vi "串口发送.vi"() -> ()   [LabVIEW 2017]
uses:
  <vilib>/Instr/_visa.llb/VISA Flush IO Buffer Mask.ctl
  <vilib>/Instr/_visa.llb/VISA Configure Serial Port (Instr).vi
panel:
  out "波形图表":dbl(graph)
  in  "停止":bool
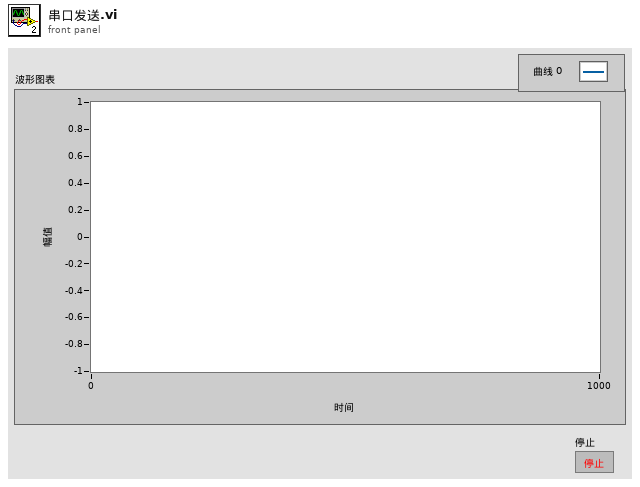
[diagram p1: front panel]
types:
  T1 = typedef "VISA Flush IO Buffer Mask.ctl" = u16
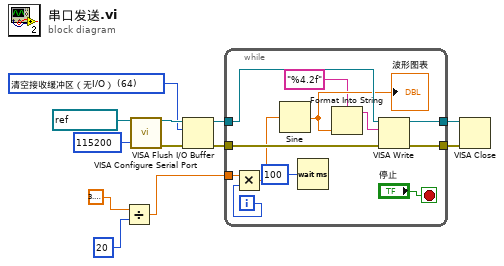
[diagram p0: block diagram]
diagram:
  w8 = T1 64 items=["清空接收缓冲区"=16, "向设备写入传输缓冲区"=32, "清空接收缓冲区（无I/O）"=64, "清空传输缓冲区"=128] ("Mask")
  n1 = Divide(x=3.141592653589793, y=20) -> (x/y=w1:dbl)
  n2 = call-poly "VISA Configure Serial Port"("VISA resource name"=refnum<visa-resource-name> "COM1", "baud rate (9600)"=u32 115200) -> ("VISA resource name out"=w12:refnum<visa-resource-name>, "error out"=w11:errorcluster)  [unwired: 12 in]
  n3 = VISA Flush I/O Buffer(VISA resource name=w12, mask (16)=w8, error in (no error)=w11) -> (VISA resource name out=w10:refnum<visa-resource-name>, error out=w9:errorcluster)
  n4 = while {
    tunnel: w10 -> [w24]
    tunnel: w9 -> [w23]
    tunnel: [w22] -> w6
    tunnel: [w21] -> w5
    tunnel: w1 -> [w17]
    i -> [w18]
    stop <- "停止" stop-if-true
    n5 = Multiply(x=w17, y=w18) -> (x*y=w16:dbl)
    n6 = Sine(x=w16) -> (sin(x)=w15:dbl)
    "波形图表" <- w15
    n7 = Wait (ms)(milliseconds to wait=u32 100 ("等待时间（毫秒）")) -> ()  [unwired: 1 out]
    n8 = Format Into String(format string="%4.2f" ("格式字符串"), w15) -> (resulting string=w14:string)  [unwired: 2 in, 1 out]
    n9 = VISA Write(VISA resource name=w24, write buffer=w14, error in (no error)=w23) -> (VISA resource name out=w22:refnum<visa-resource-name>, error out=w21:errorcluster)  [unwired: 1 out]
  }
  n10 = VISA Close(VISA resource name=w6, error in (no error)=w5) -> ()  [unwired: 1 out]
